vi "ECS - System - Exec Info.vi"   [LabVIEW 2015, in "ECS-RT.lvlib"]
uses:
  ECS-RT.lvlib
  <vilib>/NI_Real-Time Target Support.lvlib
  <resource>/objmgr/nisysapi.rc
types:
  T1 = typedef "NI_Real-Time Target Support.lvlib/RT CPU Load.ctl" = cluster{"Total (%)":dbl, "Time Critical (%)":dbl, "Timed Structures (%)":dbl, "High (%)":dbl, "Above Normal (%)":dbl, "Normal (%)":dbl, "Background (%)":dbl, "Idle (%)":dbl, "ISR (%)":dbl}
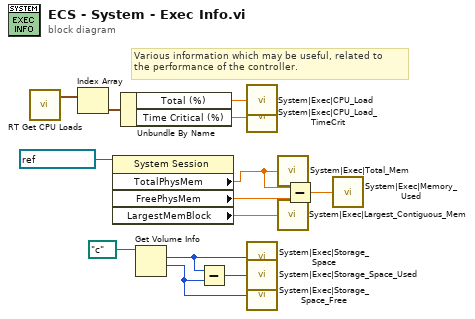
[diagram p0: block diagram]
diagram:
  # "Various information which may be useful, related to\nthe performance of the controller."
  n1 = call <vilib>:"RT Get CPU Loads.vi"() -> ("CPU loads"=w2:T1[])  [unwired: 10 in, 1 out]
  n2 = Index Array(array=w2) -> (element=w3:T1)  [unwired: 1 in]
  n3 = property class="System Session"(reference=refnum<k21> "localhost" ("System Session")) -> ("TotalPhysMem"=w7:dbl, "FreePhysMem"=w8:dbl, "LargestMemBlock"=w9:dbl)  [unwired: 1 in, 2 out]
  n4 = Unbundle By Name(w3) -> ("Total (%)"=w4:dbl, "Time Critical (%)"=w5:dbl)
  n5 = Get Volume Info(11:path "c:/" ("path")) -> (1:w13:i64, 2:w11:i64)  [unwired: 1 in, 4 out]
  n6 = Subtract(x=w11, y=w13) -> (x-y=w12:i64)
  n7 = call "System|Exec|CPU_Load"("Value"=w4) -> ()
  n8 = call "System|Exec|CPU_Load_TimeCrit"("Value"=w5) -> ()
  n9 = call "System|Exec|Storage_Space"("Value"=w11) -> ()
  n10 = call "System|Exec|Storage_Space_Used"("Value"=w12) -> ()
  n11 = call "System|Exec|Storage_Space_Free"("Value"=w13) -> ()
  n12 = call "System|Exec|Total_Mem"("Value"=w7) -> ()
  n13 = call "System|Exec|Largest_Contiguous_Mem"("Value"=w9) -> ()
  n14 = Subtract(x=w7, y=w8) -> (x-y=w1:dbl)
  n15 = call "System|Exec|Memory_Used"("Value"=w1) -> ()
